vi "Self Configure.vi"(8 "error in":errorcluster, 11 "SL_SC in":refnum<class "SL_SC.lvclass">) -> (0 "error out":errorcluster, 3 "SL_SC out":refnum<class "SL_SC.lvclass">)   [LabVIEW 2019, in "SL_SC.lvlib" / "SL_SC.lvclass"]
uses:
  Library/SL_SC.lvclass
  Custom Controls/Configuration Keys.ctl
  builds/Instruments/DIG_IO.lvlibp/Library/DIG_IO.lvclass
  builds/Tools/Config.lvlibp/Config.lvclass
  C:/Users/Public/Documents/Development/builds/Tools/Config.lvlibp/Config.lvclass
panel:
  in  "Configuration Keys":T1
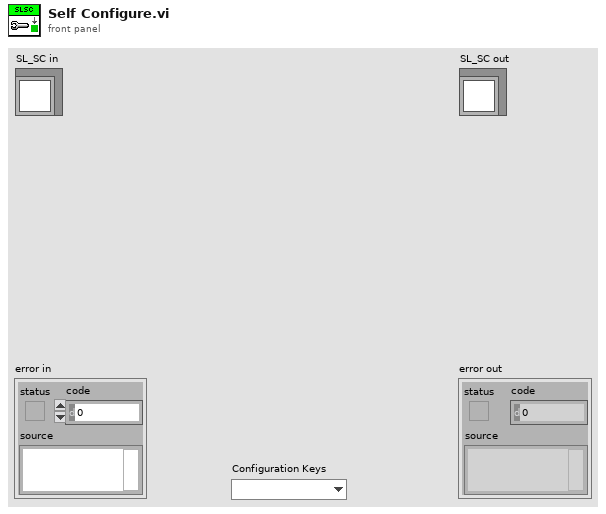
[diagram p1: front panel]
types:
  T1 = typedef "SL_SC.lvlib/SL_SC.lvclass/Configuration Keys.ctl" = enum16{""}
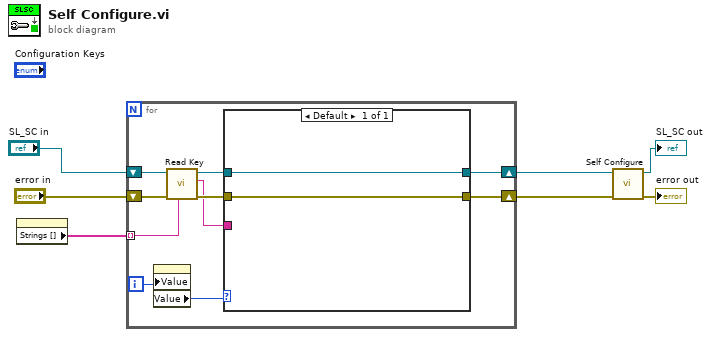
[diagram p0: block diagram]
diagram:
  n1 = property on="Configuration Keys" class="Enum (strict)"() -> ("Strings []"=w5:string[])  [unwired: 2 in, 2 out]
  n2 = for {
    tunnel: w5 -> [w13] mode=indexing
    shift-right: [w10] -> w2
    shift-left: "SL_SC in" -> [w16]
    shift-right: [w9] -> w1
    shift-left: "error in" -> [w12]
    i -> [w17]
    n3 = property on="Configuration Keys" class="Enum (strict)"("Value"=w17) -> ("Value"=w15:T1)  [unwired: 2 in, 2 out]
    n4 = call "Read Key.vi"("Key Name"=w13, "error in"=w12, "Config in"=w16) -> ("error out"=w11:errorcluster, "Key Value"=w8:string, "Config out"=w14:refnum<class "SL_SC.lvclass">)  [unwired: 6 in]
    n5 = case shown="Default" w15 {
      tunnel: w14 -> [w19]
      tunnel: w11 -> [w18]
      tunnel: [w19] -> w10
      tunnel: [w18] -> w9
      tunnel: w8 -> [_]
      frame Default {
      }
    }
  }
  n6 = call-parent "Self Configure.vi"("error in"=w1, "DIG_IO in"=w2) -> ("error out"=→"error out":errorcluster, "DIG_IO out"=→"SL_SC out":refnum<class "SL_SC.lvclass">)  [unwired: 8 in]
